vi "osq_save.vi"(8 "error in (no error)":errorcluster, 10 "SEQs":T1[](array[typedef]), 11 "Save":path=path "C:/Users/Adam/Desktop/test.json") -> (0 "error out":errorcluster, 3 "json File Path(duplicate)":path)   [LabVIEW 2015, in "oskar_tools.lvlib"]
uses:
  oskar_tools.lvlib
  seq_line.ctl
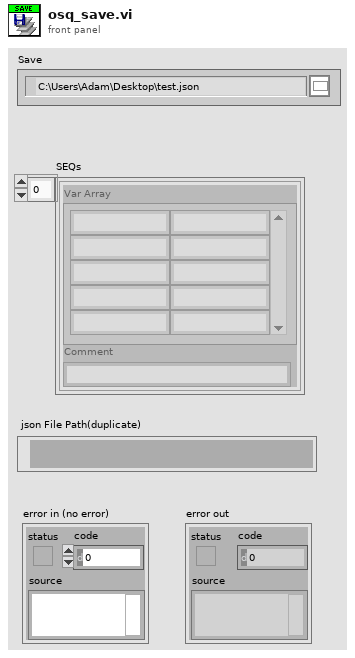
[diagram p1: front panel]
types:
  T1 = typedef "oskar_tools.lvlib/seq_line.ctl" = cluster{"Var Array":string[][], "Comment":string}
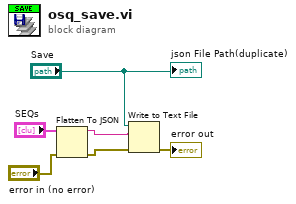
[diagram p0: block diagram]
diagram:
  n1 = Flatten To JSON(anything="SEQs", error in (no error)="error in (no error)") -> (JSON string=w5:string, 11:w2:errorcluster)  [unwired: 1 in]
  n2 = Write to Text File(file (use dialog)="Save", text=w5, error in=w2) -> (error out=→"error out":errorcluster)  [unwired: 1 in, 2 out]
  "json File Path(duplicate)" <- "Save"
